vi "PassOrFail (SubVI).vi"(5 "Test#":string, 6 "String Res":string, 7 "index (row)":i32, 8 "error in (no error)":errorcluster, 9 "Data in":dbl format="%#_13g", 10 "Pass?Fail":bool, 11 "Table in":refnum<vi>) -> (0 "error out":errorcluster)   [LabVIEW 2017]
uses:
  <vilib>/Utility/miscctls.llb/LVRowAndColumnTypeDef.ctl
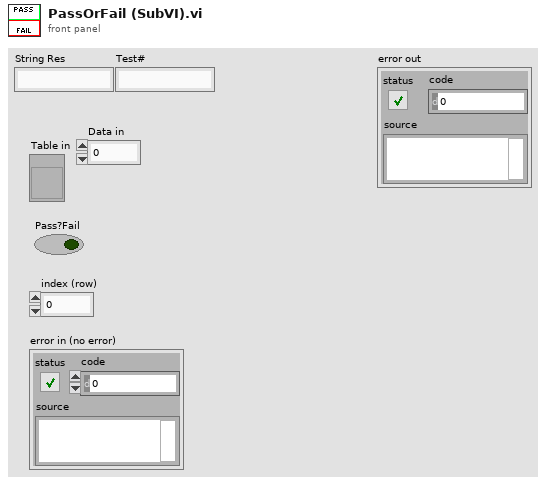
[diagram p1: front panel]
types:
  T1 = typedef "LVRowAndColumnTypeDef.ctl" = cluster{"Row":i32, "Column":i32}
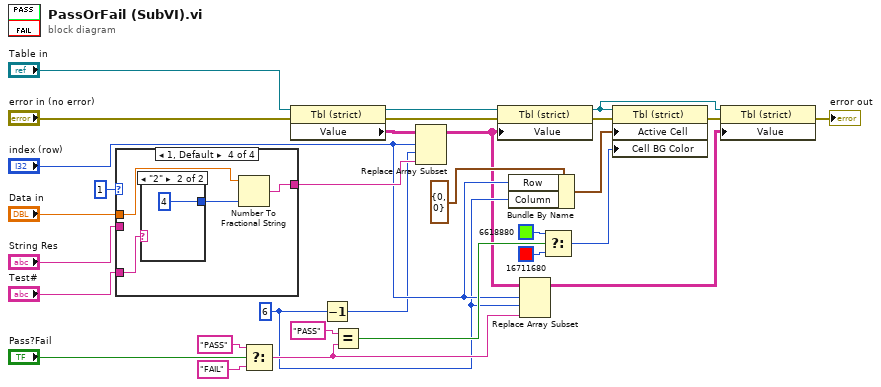
[diagram p0: block diagram]
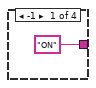
[diagram p2: hidden frame]
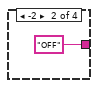
[diagram p3: hidden frame]
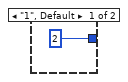
[diagram p5: hidden frame]
diagram:
  w7 = 6 ("disabled index (col)")
  n1 = case shown="1, Default" i8 1 {
    tunnel: ["ON" "OFF" w33 w37] -> w9
    tunnel: "Data in" -> [_ _ _ w35]
    tunnel: "String Res" -> [_ _ w33 _]
    tunnel: "Test#" -> [_ _ _ w34]
    frame -1 {
    }
    frame -2 {
    }
    frame -3 {
    }
    frame 1, Default {
      n2 = case shown="\"2\"" w34 {
        tunnel: [i16 2 ("precision (6)") i16 4 ("precision (6)")] -> w36
        frame "1", Default {
        }
        frame "2" {
        }
      }
      n3 = Number To Fractional String(number=w35, precision (6)=w36) -> (F-format string=w37:string)  [unwired: 2 in]
    }
  }
  n4 = Select(t="PASS" ("x"), s="Pass?Fail", f="FAIL" ("x")) -> (s? t:f=w27:string)
  n5 = property class="Tbl (strict)"(reference="Table in", error in="error in (no error)") -> (reference out=w11:refnum<vi>, error out=w12:errorcluster, "Value"=w15:string[][])
  n6 = Decrement(x=w7) -> (x-1=w6:i32)
  n7 = Equal?(x="PASS", y=w27) -> (x = y?=w17:bool)
  n8 = Replace Array Subset(array=w15, new element=w9, index (row)="index (row)", index (col)=w6) -> (w2:string[][])
  n9 = property class="Tbl (strict)"(reference=w11, error in=w12, "Value"=w2) -> (reference out=w10:refnum<vi>, error out=w24:errorcluster)
  n10 = Bundle By Name(cluster=T1 {"Row"=0, "Column"=0} ("Active Cell:Active Cell"), "Row"="index (row)", "Column"=w7) -> (w30:T1)
  n11 = Replace Array Subset(array=w2, new element=w27, index (row)="index (row)", index (col)=w7) -> (w22:string[][])
  n12 = Select(t=u32 6618880, s=w17, f=u32 16711680) -> (s? t:f=w21:u32)
  n13 = property class="Tbl (strict)"(reference=w10, error in=w24, "Active Cell"=w30, "Cell BG Color"=w21) -> (error out=w23:errorcluster)  [unwired: 1 out]
  n14 = property class="Tbl (strict)"(reference=w10, error in=w23, "Value"=w22) -> (error out=→"error out":errorcluster)  [unwired: 1 out]
